vi "Impedance.vi"(11 "file path (dialog if empty)":path) -> (0 "Abs Amplitude":dbl, 1 "Phase (deg)":dbl, 2 "Flow Freq (Hz)":dbl format="%.2p", 3 "Pressure Amp (mmHg)":dbl format="%.2p")   [LabVIEW 2018]
uses:
  <vilib>/Utility/file.llb/Read Delimited Spreadsheet (DBL).vi
  <vilib>/measure/matone.llb/Extract Single Tone Information 1 Chan.vi
  <vilib>/express/express analysis/Spectral/Block/exnSpectralBlock spectral measurements RMS poly.vi
  <vilib>/express/express analysis/Spectral/Block/exnSpectralBlock spectral measurements RMS WFM.vi
  <vilib>/express/express analysis/Spectral/XNode/ExpressSpectralMeasurementsBlockNode.xnode
  <vilib>/measure/NI_MAPro.lvlib
panel:
  out "Pressure Freq (Hz)":dbl format="%.2p"
  out "FFT - Pressure":cluster{"f0":dbl, "df":dbl, "magnitude":dbl[]}(graph)
  out "Flow Amp (mL/sec)":dbl format="%.2p"
  out "FFT - Flow":cluster{"f0":dbl, "df":dbl, "magnitude":dbl[]}(graph)
  out "Flow":cluster{"all rows":dbl[], "all rows":dbl[]}(graph)
  out "Pressure":cluster{"all rows":dbl[], "all rows":dbl[]}(graph)
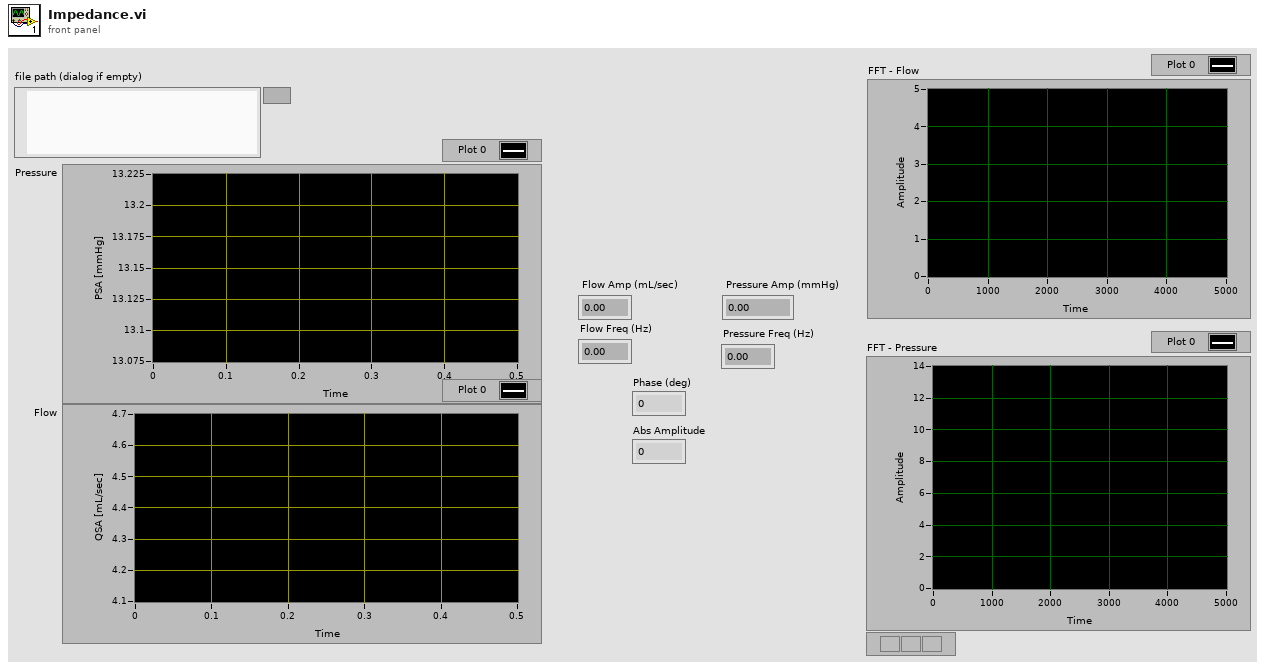
[diagram p1: front panel]
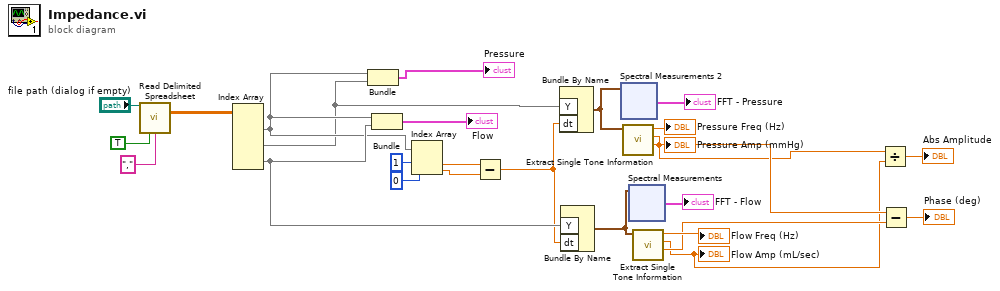
[diagram p0: block diagram]
diagram:
  n1 = call-poly <vilib>:"Read Delimited Spreadsheet.vi"("file path (dialog if empty)"="file path (dialog if empty)", "transpose? (F)"=TRUE, "delimiter (\\t)"="," ("delimiter (\\t)")) -> ("all rows"=w23:dbl[][])  [unwired: 7 in, 5 out]
  n2 = Index Array(array=w23) -> (element #1=w16:dbl[], element #2=w10:dbl[], element #3=w20:dbl[])  [unwired: 6 in]
  n3 = Bundle("all rows"=w16, "all rows"=w10) -> (→"Pressure":cluster{"all rows":dbl[], "all rows":dbl[]})  [unwired: 1 in]
  n4 = Bundle("all rows"=w16, "all rows"=w20) -> (→"Flow":cluster{"all rows":dbl[], "all rows":dbl[]})  [unwired: 1 in]
  n5 = Index Array(array=w16, index #1=1 ("index"), index #2=0 ("index")) -> (element #1=w13:dbl, element #2=w12:dbl)
  n6 = Subtract(x=w13, y=w12) -> (x-y=w11:dbl)
  n7 = Bundle By Name("Y"=w10, "dt"=w11) -> (w8:waveform(dbl))  [unwired: 1 in]
  n8 = Bundle By Name("Y"=w20, "dt"=w11) -> (w18:waveform(dbl))  [unwired: 1 in]
  n9 = xnode ("Spectral Measurements 2")("Signals"=w8) -> ("FFT - (RMS)"=→"FFT - Pressure":cluster{"f0":dbl, "df":dbl, "magnitude":dbl[]})  [unwired: 1 in, 2 out]
  n10 = call-poly <vilib>:"Extract Single Tone Information.vi"("time signal in"=w8) -> ("detected phase (deg)"=w6:dbl, "detected amplitude"=w3:dbl, "detected frequency"=→"Pressure Freq (Hz)":dbl)  [unwired: 5 in, 3 out]
  "Pressure Amp (mmHg)" <- w3
  n11 = xnode ("Spectral Measurements")("Signals"=w18) -> ("FFT - (RMS)"=→"FFT - Flow":cluster{"f0":dbl, "df":dbl, "magnitude":dbl[]})  [unwired: 1 in, 2 out]
  n12 = call-poly <vilib>:"Extract Single Tone Information.vi"("time signal in"=w18) -> ("detected phase (deg)"=w5:dbl, "detected amplitude"=w2:dbl, "detected frequency"=→"Flow Freq (Hz)":dbl)  [unwired: 5 in, 3 out]
  "Flow Amp (mL/sec)" <- w2
  n13 = Divide(x=w3, y=w2) -> (x/y=→"Abs Amplitude":dbl)
  n14 = Subtract(x=w6, y=w5) -> (x-y=→"Phase (deg)":dbl)
